vi "Read_OPC_Model_SN.vi"(2 "Model Type":u16 format="%x") -> (5 "Type":string, 6 "Serial Number":string, 7 "Knop":cluster{"FL":bool, "FR":bool}, 8 "Detail":string)   [LabVIEW 2017]
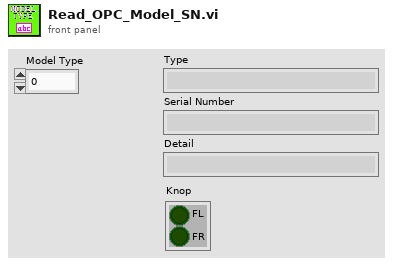
[diagram p1: front panel]
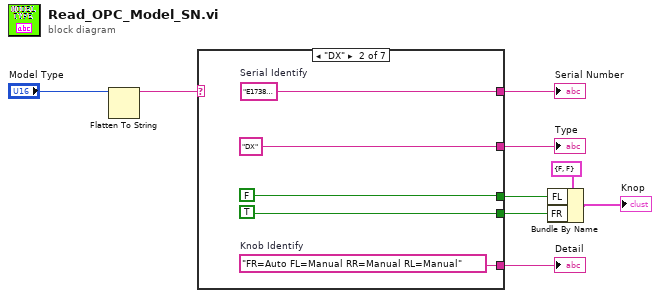
[diagram p0: block diagram]
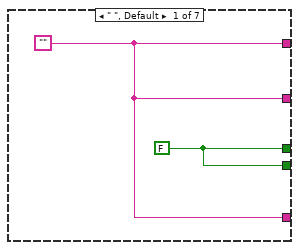
[diagram p2: hidden frame]
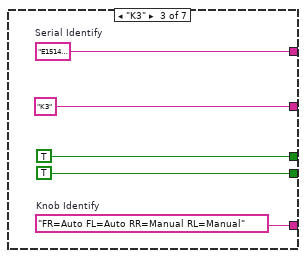
[diagram p3: hidden frame]
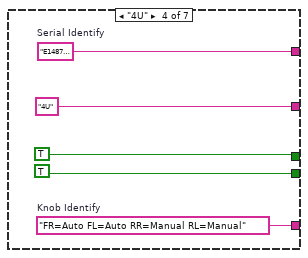
[diagram p4: hidden frame]
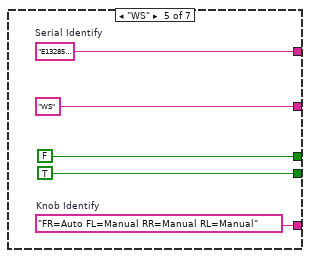
[diagram p5: hidden frame]
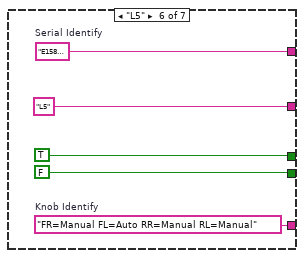
[diagram p6: hidden frame]
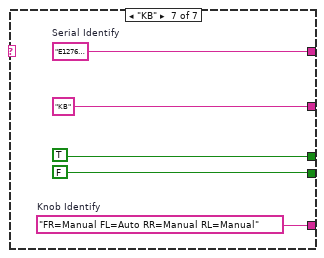
[diagram p7: hidden frame]
diagram:
  n1 = Flatten To String(anything="Model Type") -> (data string=w9:string)  [unwired: 3 in, 2 out]
  n2 = case shown="\"DX\"" w9 {
    tunnel: [w11 w16 w21 w26 w31 w36 w41] -> w8
    tunnel: [w11 "DX" "K3" "4U" "WS" "L5" "KB"] -> w6
    tunnel: [w11 w14 w19 w24 w29 w34 w39] -> w5
    tunnel: [w10 FALSE TRUE TRUE FALSE TRUE TRUE] -> w2
    tunnel: [w10 TRUE TRUE TRUE TRUE FALSE FALSE] -> w1
    frame " ", Default {
      w10 = FALSE
      w11 = ""
    }
    frame "DX" {
      w14 = "FR=Auto FL=Manual RR=Manual RL=Manual"  # Knob Identify
      w16 = "E173839 254016PA3A"  # Serial Identify
    }
    frame "K3" {
      w19 = "FR=Auto FL=Auto RR=Manual RL=Manual"  # Knob Identify
      w21 = "E151441 254016PA2A"  # Serial Identify
    }
    frame "4U" {
      w24 = "FR=Auto FL=Auto RR=Manual RL=Manual"  # Knob Identify
      w26 = "E148761 254016PA1A"  # Serial Identify
    }
    frame "WS" {
      w29 = "FR=Auto FL=Manual RR=Manual RL=Manual"  # Knob Identify
      w31 = "E132857 254016LA1A"  # Serial Identify
    }
    frame "L5" {
      w34 = "FR=Manual FL=Auto RR=Manual RL=Manual"  # Knob Identify
      w36 = "E158515 254016LA2A"  # Serial Identify
    }
    frame "KB" {
      w39 = "FR=Manual FL=Auto RR=Manual RL=Manual"  # Knob Identify
      w41 = "E127652 254016LA0A"  # Serial Identify
    }
  }
  "Serial Number" <- w8
  "Type" <- w6
  "Detail" <- w5
  n3 = Bundle By Name(cluster=cluster{"FL":bool, "FR":bool} {"FL"=FALSE, "FR"=FALSE} ("Knop"), "FL"=w2, "FR"=w1) -> (→"Knop":cluster{"FL":bool, "FR":bool})
